vi "Initialise globals.vi"(8 "error in (no error)":errorcluster) -> (0 "error out":errorcluster)   [LabVIEW 2020]
uses:
  Peripherals Control/Shutter/Typedefs/Shutter state.ctl
  User Interface/Visualisation/Functional Imaging Viewer/Typedefs/Get-Set-Clear Control.ctl
  Typedefs/Read Write Enum.ctl
  Typedefs/HW config states enum.ctl
  Typedefs/Functional global standard states.ctl
  Typedefs/AVI implementation enum.ctl
  Typedefs/Save-Load enum.ctl
  User Interface/Globals/gl_Windows Ctrl refs.vi
  General Globals.vi
  User Interface/Globals/gl_Funct imaging UI.vi
  Configuration code/Calibration/Globals/gl_Calibration globals.vi
  User Interface/Windows/System config window/Globals/Sys Config window globals.vi
  Peripherals Control/XYZ Stage/Globals/gl_XYZStage globals.vi
  gl_UI Ctrl Refs.vi
  Typedefs/test_fpga_control.ctl
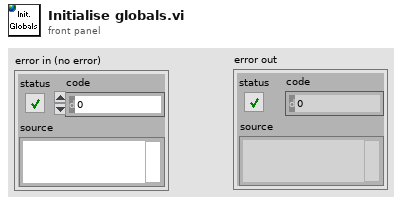
[diagram p1: front panel]
types:
  T1 = typedef "Shutter state.ctl" = enum16{"Closed/Disabled", "Open/Enabled"}
  T2 = enum16{"Initialise", "Load from file", "Save to file", "Read", "Write"}
  T3 = typedef "Functional global standard states.ctl" = enum16{"Initialise", "Read", "Write", "Load", "Save", "Clear"}
  T4 = typedef "Read Write Enum.ctl" = enum16{"Read", "Write"}
  T5 = typedef "Get-Set-Clear Control.ctl" = enum16{"Get", "Set", "Clear"}
  T6 = typedef "Save-Load enum.ctl" = enum16{"Save to file", "Load from file", "Compare from file", "Save Backup"}
  T7 = typedef "AVI implementation enum.ctl" = enum16{"AVI1", "AVI2"}
  T8 = enum16{"Write Red AVI", "Write Green AVI", "Write AVI mode"}[]
  T9 = typedef "HW config states enum.ctl" = enum16{"Load from file", "Save to file", "Save backup", "Write all", "Read all", "Write XY stage settings", "Write DAQ FPGA settings", "Write Control FPGA settings", "Write Phys Channels", "Write System Config", "Write HW Config", "Save System Config", "Save HW Config", "Clear", "Compare from file"}
  T10 = typedef "test_fpga_control.ctl" = cluster{"x_offset_host":fxp<+/-,16,8>, "y_offset_host":fxp<+/-,16,8>, "use host offset":bool, "Set_Ref_Centroid":bool, "OldChirpCode":bool, "use array of offsets":bool, "x_offset_host array":fxp<+/-,16,8>[], "y_offset_host array ":fxp<+/-,16,8>[], "use host offset Z":bool, "swap Z":bool, "z_offset_host ":fxp<+/-,16,8>}
  T11 = typedef "Calibration config.ctl" = cluster{"Current Objective":string, "Objective Settings":T12[], "PreChirper Values Preset ?":bool, "PreChirper Settings":T13[], "PreChirper Constants":T14}
  T12 = typedef "Objective Config.ctl" = cluster{"Name":string, "Sum X":dbl, "Sum Y":dbl, "Diff X":dbl, "Diff Y":dbl, "Distortion Correction":dbl, "Z_norm to um_scaling":dbl, "X_norm to um_scaling":dbl, "Calibrated Wavelength":dbl}
  T13 = typedef "Prechirper Cal Config.ctl" = cluster{"Wavelength":i32, "Prism 1":i32, "Prism 2":i32}
  T14 = typedef "PreChirper constants.ctl" = cluster{"a 1":i32, "b 1":i32, "c 1":i32, "a 2":i32, "b 2":i32, "c 2":i32, "lmin":i32, "lmax":i32}
  T15 = typedef "UI ctrl refs cluster.ctl" = cluster{"Top level VI path":path, "Top level VI ref":refnum<vi>, "User menu ref":refnum<k9>, "Sub Panel control":refnum<vi>, "Imaging Param Tab":refnum<vi>, "Occurrence-Start drivers":refnum<k4>, "Occurrence-Speed logging initialised":refnum<k4>, "Occurrence-XYZ stage initialised":refnum<k4>, "Exit button":refnum<vi>, "Status ind":refnum<vi>, "Set as origin":refnum<vi>, "Speed Logging":refnum<vi>, "Time Lapse":refnum<vi>, "Live Imaging":refnum<vi>, "AOL Z Stack":refnum<vi>, "Motor Z Stack":refnum<vi>, "Funct Acq button":refnum<vi>, "Hard Shutter":refnum<vi>, "Virtual Shutter":refnum<vi>, "Laser Power":refnum<vi>, "AOL Mode":refnum<vi>, "Frame Size":refnum<vi>, "Field of View":refnum<vi>, "Dwell Time":refnum<vi>, "Zoom":refnum<vi>, "AOL Z":refnum<vi>, "Objective":refnum<vi>, "Axis":refnum<vi>, "Paths & Names":refnum<vi>, "Experiment folder path (ind.)":refnum<vi>, "Last State (Ind.)":refnum<vi>, "Averages":refnum<vi>, "Angle (degrees)":refnum<vi>, "X centre":refnum<vi>, "Y centre":refnum<vi>, "Plane Mode":refnum<vi>, "# Planes":refnum<vi>, "Z Start":refnum<vi>, "Z Stop":refnum<vi>, "Z Step":refnum<vi>, "PMT 1":refnum<vi>, "PMT 2":refnum<vi>, "Stage XYZ Position":refnum<vi>, "Pockels@Z Start":refnum<vi>, "Pockels@Z Stop":refnum<vi>, "Obtain Z Start":refnum<vi>, "Obtain Z Stop":refnum<vi>, "Live stim.trig.period":refnum<vi>, "Live stim.trig.enable":refnum<vi>, "Movement Correction":refnum<vi>, "Load Reference Image":refnum<vi>, "XY Stage Move":refnum<vi>, "MovCor Cluster":refnum<vi>, "RefDAQParam":refnum<vi>, "Funct. Acq. Pockels Modulation":refnum<vi>, "Ref Laser Power":refnum<vi>, "Enable Video Recording":refnum<vi>, "Video Record-Live Imaging":refnum<vi>, "Video Record-Funct acq":refnum<vi>, "Reference Source":refnum<vi>, "AOL Z-stack Chirps Ready (ind)":refnum<vi>, "Target time between mov.cor. ref triggers (ms)":refnum<vi>, "Funct. Acq. Ref frame save":refnum<vi>, "Tracking button":refnum<vi>, "Show ref plots window":refnum<vi>, "Center freq ind (nm)":refnum<vi>, "Pickup mode (ind)":refnum<vi>, "Logging queue (ind)":refnum<vi>, "Back aperture power (ind.)":refnum<vi>, "Power after objective (ind.)":refnum<vi>, "Switch user":refnum<vi>, "Ls1 Conn. Status":refnum<vi>, "Ls1Tuning Status":refnum<vi>, "Ls1 Faults":refnum<vi>, "Ls1 Connection":refnum<vi>, "Ls1 Mode":refnum<vi>, "Ls1 POWER [mW]":refnum<vi>, "Ls1Shutter":refnum<vi>, "Ls1 Wavelength":refnum<vi>, "Ls1 Note":refnum<vi>, "Ls1 Confirm Wav":refnum<vi>, "Ls1 PreChrp Prism1":refnum<vi>, "Ls1 PreChrp Prism2":refnum<vi>, "Ls1 wav top Ind":refnum<vi>, "Ls1 power top Ind":refnum<vi>, "Ls1 Pump peak Hold":refnum<vi>, "Ls1 Status Ind":refnum<vi>, "Ls1 wav cancel":refnum<vi>, "Experiment Type":refnum<vi>, "Biology Information":refnum<vi>, "Camera recording status":refnum<vi>}
  T16 = typedef "Ref DAQ Param.ctl" = cluster{"Full Frame Size":u16, "Ref Field of View":sgl, "Ref Zoom":i8, "Ref_dwellTime":sgl, "Ref X-pixels-per-line(Npxr)":i16, "Ref Y-lines-per-image(Npyr)":i16, "Ref Z-lines-per-image":i16, "Ignore Z lines":i16, "Ref Scan Cycles":i32, "Ref threshold XY":u16, "Ref threshold Z":u16, "Ref average XY":u16, "Ref Average  Z":u16, "Proportional_scale":fxp<+,16,2>, "Integral_scale":fxp<+/-,16,12>, "Proportional_scale Z":fxp<+,16,2>, "Integral_scale Z":fxp<+/-,16,12>, "Diff_threshold":fxp<+,16,2>, "Diff_threshold _z":fxp<+,16,2>, "Sliding Average":bool, "Ref count reset enabled":bool}
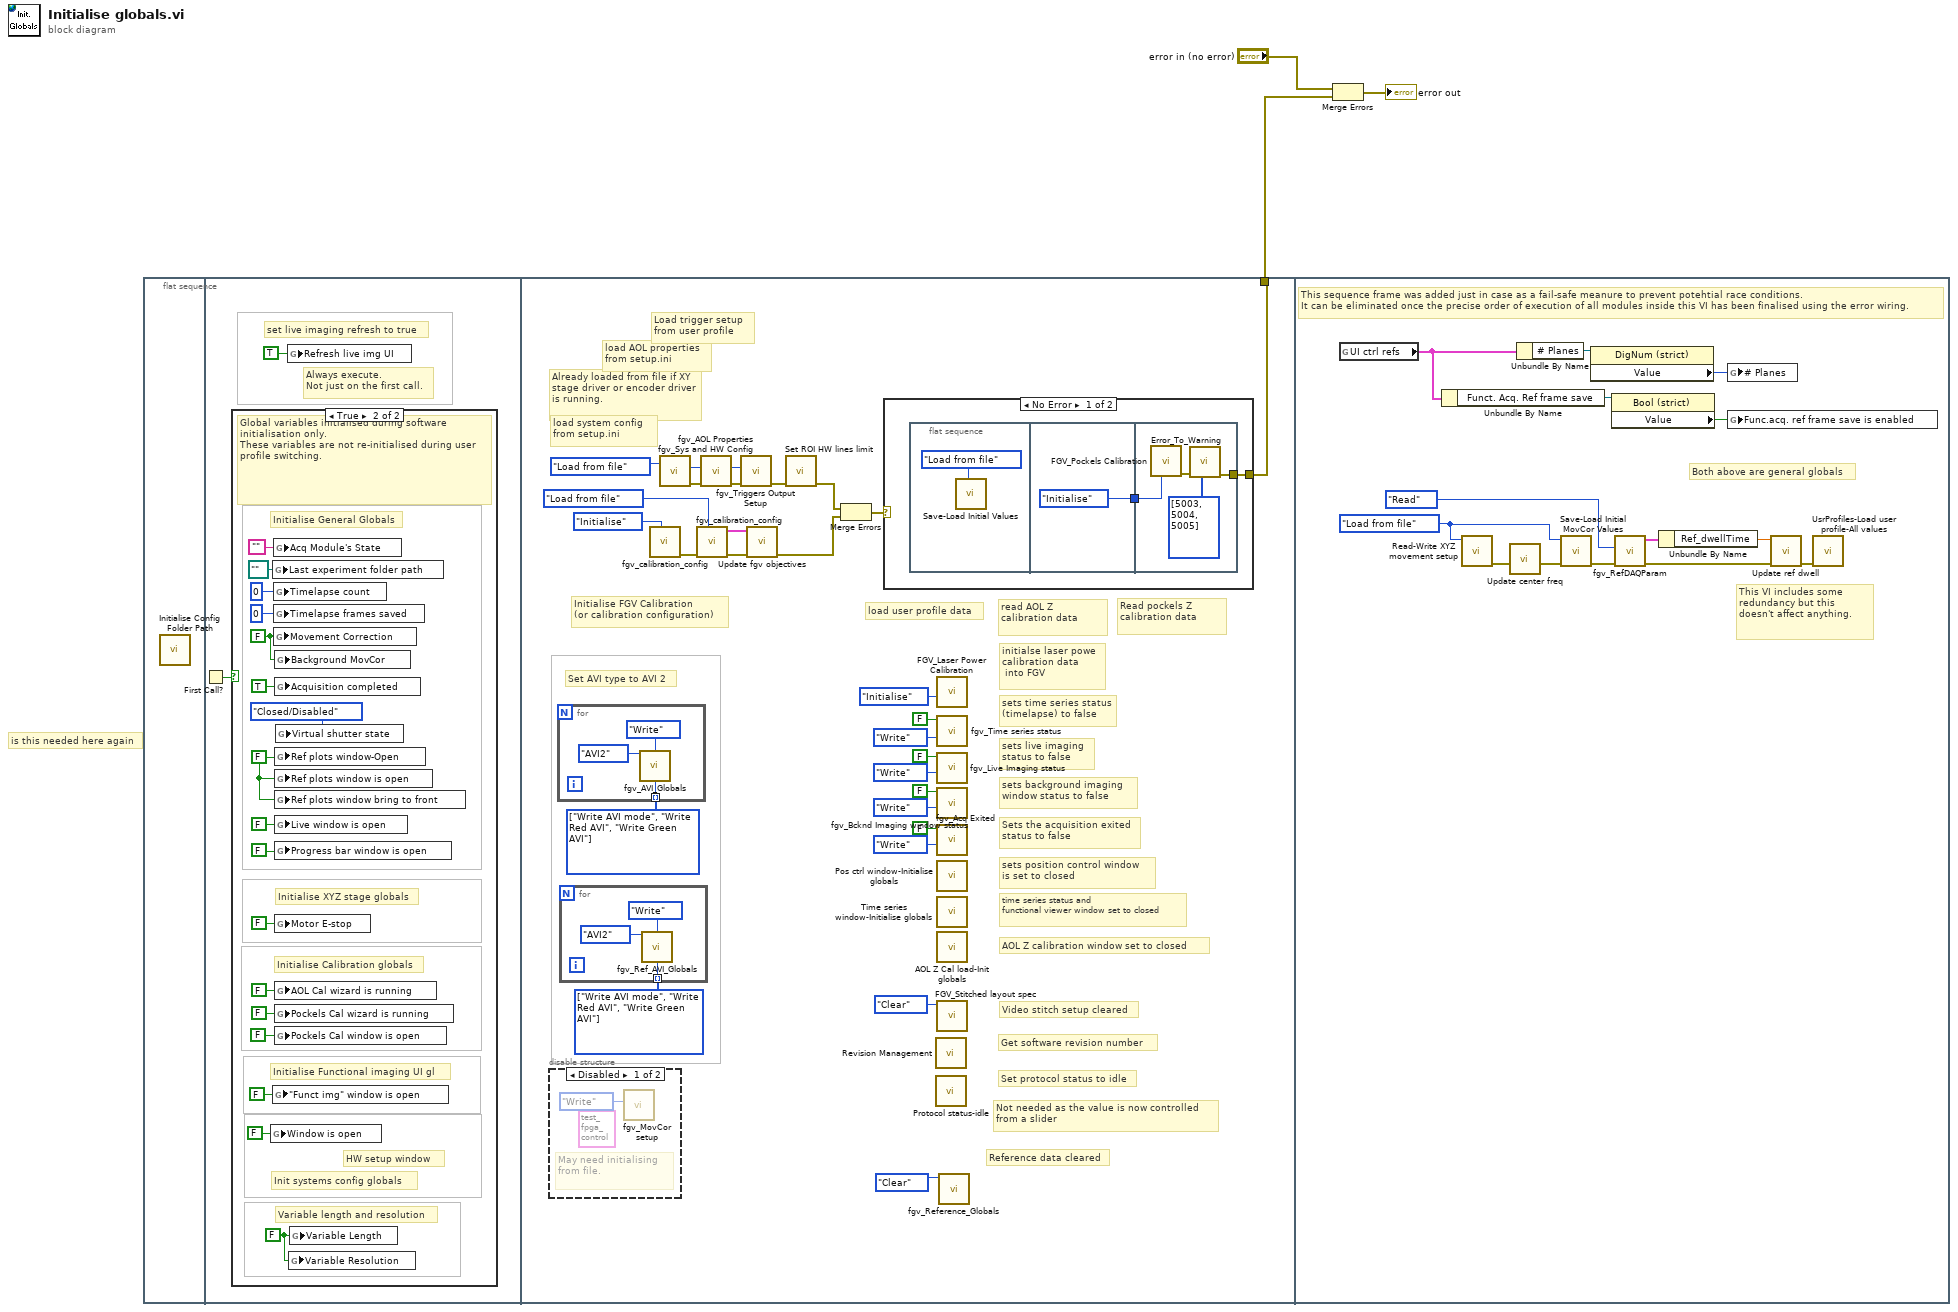
[diagram p0: block diagram]
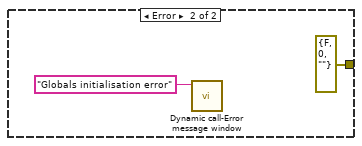
[diagram p3: hidden frame]
diagram:
  # "is this needed here again"
  n1 = flat-sequence {
    tunnel: [w34] -> w3
    frame #0 {
      n2 = call "Initialise Config Folder Path.vi"() -> ()  [unwired: 9 in, 3 out]
    }
    frame #1 {
      # "set live imaging refresh to true"
      # "Always execute.\nNot just on the first call."
      n3 = First Call?() -> (First Call?: T/F=w5:bool)
      n4 = case shown="True" w5 {
        frame False {
        }
        frame True {
          w6 = FALSE ("Variable Length")
          w11 = FALSE ("Movement Correction")
          w22 = FALSE ("Bring to front")
          # "Variable length and resolution"
          # "Init systems config globals"
          # "Initialise Functional imaging UI gl"
          # "Initialise Calibration globals"
          # "Initialise XYZ stage globals"
          # "Initialise General Globals"
          # "HW setup window"
          # "Global variables initialised during software initialisation only.\nThese variables are not re-initialised during user profile switching."
          n5 = global write "Sys Config window globals.vi" "Window is open"(FALSE ("Bring to front")) -> ()
          n6 = global write "General Globals.vi" "Last experiment folder path"(path "" ("Last experiment folder path")) -> ()
          n7 = global write "gl_Funct imaging UI.vi" "\"Funct img\" window is open"(FALSE ("\"Funct img\" window is open")) -> ()
          n8 = global write "General Globals.vi" "Acq Module's State"("" ("Acq Module's State")) -> ()
          n9 = global write "General Globals.vi" "Timelapse count"(u32 0 ("Timelapse count")) -> ()
          n10 = global write "General Globals.vi" "Timelapse frames saved"(u32 0 ("Timelapse frames saved")) -> ()
          n11 = global write "General Globals.vi" "Movement Correction"(w11) -> ()
          n12 = global write "General Globals.vi" "Background MovCor"(w11) -> ()
          n13 = global write "General Globals.vi" "Acquisition completed"(TRUE ("Acquisition completed")) -> ()
          n14 = global write "General Globals.vi" "Ref plots window-Open"(w22) -> ()
          n15 = global write "General Globals.vi" "Ref plots window is open"(w22) -> ()
          n16 = global write "General Globals.vi" "Ref plots window bring to front"(w22) -> ()
          n17 = global write "General Globals.vi" "Live window is open"(FALSE ("Live window running")) -> ()
          n18 = global write "General Globals.vi" "Progress bar window is open"(FALSE ("Progress bar window is open")) -> ()
          n19 = global write "gl_XYZStage globals.vi" "Motor E-stop"(FALSE ("Motor E-stop")) -> ()
          n20 = global write "gl_Calibration globals.vi" "AOL Cal wizard is running"(FALSE ("Motor Z Cal wizard is running")) -> ()
          n21 = global write "gl_Calibration globals.vi" "Pockels Cal wizard is running"(FALSE ("Pockels Cal wizard is running")) -> ()
          n22 = global write "gl_Calibration globals.vi" "Pockels Cal window is open"(FALSE ("Pockels Cal window is open")) -> ()
          n23 = global write "General Globals.vi" "Virtual shutter state"(Shutter_state."Closed/Disabled" ("Virtual shutter state")) -> ()
          n24 = global write "General Globals.vi" "Variable Resolution"(w6) -> ()
          n25 = global write "General Globals.vi" "Variable Length"(w6) -> ()
        }
      }
      n26 = global write "gl_Windows Ctrl refs.vi" "Refresh live img UI"(TRUE ("Refresh live img UI")) -> ()
    }
    frame #2 {
      w38 = T8 [enum."Write AVI mode", enum."Write Red AVI", enum."Write Green AVI"] items=["Write Red AVI", "Write Green AVI", "Write AVI mode"]
      w37 = T8 [enum."Write AVI mode", enum."Write Red AVI", enum."Write Green AVI"] items=["Write Red AVI", "Write Green AVI", "Write AVI mode"]
      w33 = HW_config_states_enum."Load from file" ("Function")
      # "Not needed as the value is now controlled\nfrom a slider"
      # "Initialise FGV Calibration\n(or calibration configuration)"
      # "Set protocol status to idle"
      # "Get software revision number"
      # "Video stitch setup cleared"
      # "Reference data cleared"
      # "AOL Z calibration window set to closed"
      # "time series status and \nfunctional viewer window set to closed"
      # "sets position control window\nis set to closed"
      # "Sets the acquisition exited\nstatus to false"
      # "sets background imaging\nwindow status to false"
      # "sets live imaging \nstatus to false"
      # "sets time series status\n(timelapse) to false"
      # "initialse laser powe \ncalibration data\n into FGV"
      # "Set AVI type to AVI 2"
      # "Read pockels Z calibration data"
      # "read AOL Z calibration data"
      # "load user profile data"
      # "Load trigger setup \nfrom user profile"
      # "load AOL properties\nfrom setup.ini"
      # "load system config \nfrom setup.ini"
      # "Already loaded from file if XY stage driver or encoder driver is running."
      n27 = disable-structure shown="Disabled" {
        frame Disabled {
          (unwired) T10 {"x_offset_host"=0.0, "y_offset_host"=0.0, "use host offset"=FALSE, "Set_Ref_Centroid"=FALSE, "OldChirpCode"=FALSE, "use array of offsets"=FALSE, "x_offset_host array"=[], "y_offset_host array "=[], "use host offset Z"=TRUE, "swap Z"=FALSE, "z_offset_host "=0.0} ("MovCor Cluster")
          # "May need initialising from file."
          n28 = call "fgv_MovCor setup.vi"("Status"=enum16{"Initialize", "Write", "Read"}."Write") -> ()  [unwired: 9 in, 2 out]
        }
        frame Enabled {
        }
      }
      n29 = for {
        tunnel: w37 -> [w63] mode=indexing
        n30 = call "fgv_AVI_Globals.vi"("AVI mode"=AVI_implementation_enum."AVI2", "Function"=enum16{"Intialize", "Write", "Read", "Clear"}."Write", "\"Write\" sub function"=w63) -> ()  [unwired: 9 in, 4 out]
      }
      n31 = for {
        tunnel: w38 -> [w60] mode=indexing
        n32 = call "fgv_Ref_AVI_Globals.vi"("AVI mode"=AVI_implementation_enum."AVI2", "Function"=enum16{"Intialize", "Write", "Read", "Clear"}."Write", "\"Write\" sub function"=w60) -> ()  [unwired: 9 in, 4 out]
      }
      n33 = call "fgv_calibration_config.vi"("Cal config ops"=T2."Initialise") -> ("error out"=w30:errorcluster)  [unwired: 8 in, 2 out]
      n34 = call "fgv_Sys and HW Config.vi"("Function"=w33) -> ("error out"=w36:errorcluster)  [unwired: 8 in, 2 out]
      n35 = call "fgv_calibration_config.vi"("Cal config ops"=T2."Load from file", "error in (no error)"=w30) -> ("error out"=w27:errorcluster, "Config cluster OUT"=w25:T11)  [unwired: 7 in, 1 out]
      n36 = call "fgv_AOL Properties.vi"("error in (no error)"=w36, "Function"=w33) -> ("error out"=w35:errorcluster)  [unwired: 8 in, 1 out]
      n37 = call "fgv_Triggers Output Setup.vi"("error in (no error)"=w35, "Function"=w33) -> ("error out"=w24:errorcluster)  [unwired: 7 in, 2 out]
      n38 = call "Update fgv objectives.vi"("error in (no error)"=w27, "Config cluster IN"=w25) -> ("error out"=w26:errorcluster)  [unwired: 9 in]
      n39 = call "Set ROI HW lines limit.vi"("error in (no error)"=w24) -> ("error out"=w23:errorcluster)  [unwired: 10 in]
      n40 = Merge Errors(w23, w26) -> (w28:errorcluster)
      n41 = case shown="No Error" w28 {
        tunnel: [w50 errorcluster {"status"=FALSE, "code"=0, "source"=""} ("error out")] -> w34
        frame No Error {
          n42 = flat-sequence {
            tunnel: [Functional_global_standard_states."Initialise" ("Function")] -> w49
            tunnel: [w54] -> w50
            tunnel: w49 -> [w53]
            frame #0 {
              n43 = call "Save-Load Initial Values.vi"("Function"=Save-Load_enum."Load from file") -> ()  [unwired: 10 in, 1 out]
            }
            frame #1 {
            }
            frame #2 {
              n44 = call "FGV_Pockels Calibration.vi"("Function"=w53) -> ("error out"=w56:errorcluster)  [unwired: 4 in, 6 out]
              n45 = call <userlib>:"Error_To_Warning.vi"("Error Codes to be handled as warnings"=i32[] [5003, 5004, 5005], "error in"=w56) -> ("error out"=w54:errorcluster)  [unwired: 9 in]
            }
          }
        }
        frame Error {
          n46 = call "Dynamic call-Error message window.vi"("Error Message"="Globals initialisation error" ("message")) -> ()  [unwired: 10 in, 1 out]
        }
      }
      n47 = call "Revision Management.vi"() -> ()  [unwired: 11 in, 1 out]
      n48 = call "Protocol status-idle.vi"() -> ()  [unwired: 12 in]
      n49 = call "FGV_Laser Power Calibration.vi"("Function"=Functional_global_standard_states."Initialise") -> ()  [unwired: 7 in, 4 out]
      n50 = call "fgv_Time series status.vi"("Function"=Read_Write_Enum."Write", "Timelapse?"=FALSE) -> ()  [unwired: 9 in, 1 out]
      n51 = call "fgv_Live Imaging status.vi"("Function"=Read_Write_Enum."Write", "Live Imaging?"=FALSE) -> ()  [unwired: 8 in, 2 out]
      n52 = call "fgv_Bcknd Imaging window status.vi"("Function"=Read_Write_Enum."Write", "Background MovCor window is open"=FALSE) -> ()  [unwired: 8 in, 2 out]
      n53 = call "fgv_Acq Exited.vi"("Function"=Read_Write_Enum."Write", "Acquisition completed"=FALSE ("Timelapse?")) -> ()  [unwired: 8 in, 2 out]
      n54 = call "Pos ctrl window-Initialise globals.vi"() -> ()  [unwired: 12 in]
      n55 = call "Time series window-Initialise globals.vi"() -> ()  [unwired: 12 in]
      n56 = call "AOL Z Cal load-Init globals.vi"() -> ()  [unwired: 12 in]
      n57 = call "FGV_Stitched layout spec.vi"("Function"=Get-Set-Clear_Control."Clear") -> ()  [unwired: 9 in, 2 out]
      n58 = call "fgv_Reference_Globals.vi"("Function"=enum16{"Intialize", "Write", "Read", "Clear"}."Clear") -> ()  [unwired: 9 in, 2 out]
    }
    frame #3 {
      w69 = Save-Load_enum."Load from file" ("Function")
      # "Both above are general globals"
      # "This VI includes some redundancy but this doesn't affect anything."
      # "This sequence frame was added just in case as a fail-safe meanure to prevent potehtial race conditions.\nIt can be eliminated once the precise order of execution of all modules inside this VI has been finalised using the error wiring."
      n59 = global read "gl_UI Ctrl Refs.vi" "UI ctrl refs"() -> (w73:T15)
      n60 = Unbundle By Name(w73) -> ("Funct. Acq. Ref frame save"=w74:refnum<vi>)
      n61 = call "Read-Write XYZ movement setup.vi"("Function"=w69) -> ("error out"=w68:errorcluster)  [unwired: 10 in]
      n62 = call "Update center freq.vi"("error in (no error)"=w68) -> ("error out"=w70:errorcluster)  [unwired: 10 in]
      n63 = Unbundle By Name(w73) -> ("# Planes"=w79:refnum<vi>)
      n64 = call "Save-Load Initial MovCor Values.vi"("error in"=w70, "Function"=w69) -> ("error out"=w71:errorcluster)  [unwired: 9 in]
      n65 = property class="DigNum (strict)"(reference=w79) -> ("Value"=w78:u16)  [unwired: 1 in, 2 out]
      n66 = property class="Bool (strict)"(reference=w74) -> ("Value"=w72:bool)  [unwired: 1 in, 2 out]
      n67 = call "fgv_RefDAQParam.vi"("error in (no error)"=w71, "Function"=enum16{"Initialize", "Write", "Read"}."Read" ("Status")) -> ("error out"=w67:errorcluster, "RefDAQParam"=w75:T16)  [unwired: 8 in]
      n68 = Unbundle By Name(w75) -> ("Ref_dwellTime"=w77:sgl)
      n69 = global write "General Globals.vi" "# Planes"(w78) -> ()
      n70 = global write "General Globals.vi" "Func.acq. ref frame save is enabled"(w72) -> ()
      n71 = call "Update ref dwell.vi"("error in (no error)"=w67, "Ref_dwellTime"=w77) -> ("error out"=w66:errorcluster)  [unwired: 9 in]
      n72 = call "UsrProfiles-Load user profile-All values.vi"("error in"=w66) -> ()  [unwired: 10 in, 1 out]
    }
  }
  n73 = Merge Errors("error in (no error)", w3) -> (→"error out":errorcluster)
